vi "Bead Tracking Overlay matches.vi"(7 "Search Rectangle":T4, 8 "error in (no error)":errorcluster, 9 "Bead Tracking Mode":T1, 10 "Matches":T2, 11 "Image":T3) -> (0 "error out":errorcluster, 3 "Image out":T3)   [LabVIEW 2011]
doc: "This VI adds overlays to an image, to show the bead tracking results graphically."
uses:
  <vilib>/vision/Image Controls.llb/IMAQ Image.ctl
  Bead Tracking Matches.ctl
  Bead Tracking Mode.ctl
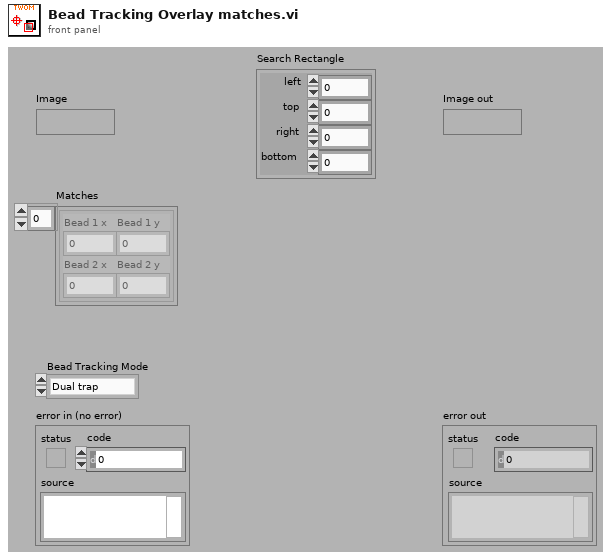
[diagram p1: front panel]
types:
  T1 = typedef "Bead Tracking Mode.ctl" = enum16{"Dual trap", "Q-trap =", "Q-trap ||", "Q-trap X", "Q-trap +", "Dual trap oO", "Single trap", "None"}
  T2 = typedef "Bead Tracking Matches.ctl" = cluster{"Bead 1 x":dbl, "Bead 1 y":dbl, "Bead 2 x":dbl, "Bead 2 y":dbl}[]
  T3 = typedef "IMAQ Image.ctl" = refnum<image>
  T4 = cluster{"left":i16, "top":i16, "right":i16, "bottom":i16}
  T5 = cluster{"Bead 1 x":dbl, "Bead 1 y":dbl, "Bead 2 x":dbl, "Bead 2 y":dbl}
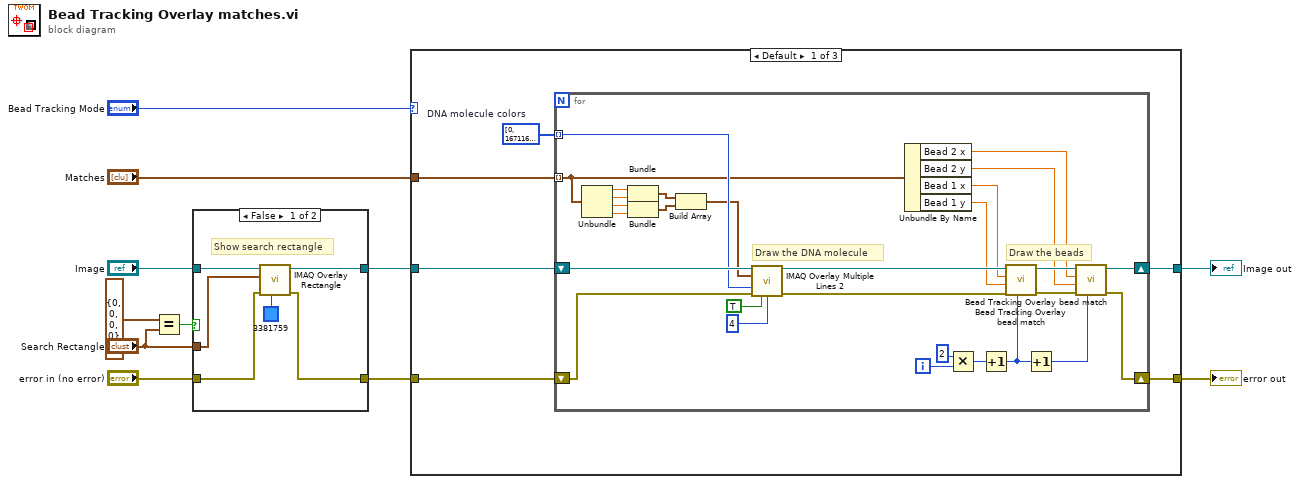
[diagram p0: block diagram]
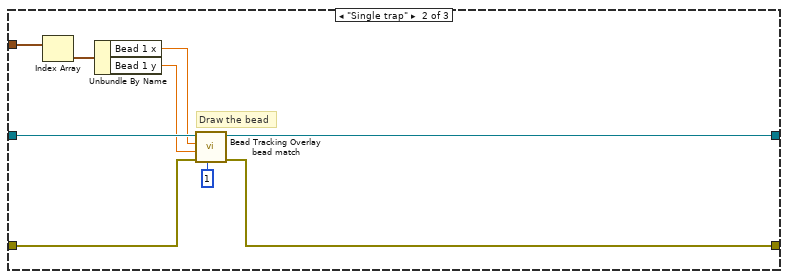
[diagram p2: hidden frame]
diagram:
  n1 = Equal?(x=T4 {"left"=0, "top"=0, "right"=0, "bottom"=0}, y="Search Rectangle") -> (x = y?=w11:bool)
  n2 = case shown="False" w11 {
    tunnel: "Image" -> [w17 w19]
    tunnel: [w16 w19] -> w6
    tunnel: "Search Rectangle" -> [w15 _]
    tunnel: "error in (no error)" -> [w14 w18]
    tunnel: [w12 w18] -> w4
    frame False {
      # "Show search rectangle"
      n3 = call "IMAQ Overlay Rectangle"("Color"=u32 3381759, "error in (no error)"=w14, "Rectangle"=w15, "Image"=w17) -> ("error out"=w12:errorcluster, "Image Out"=w16:T3)  [unwired: 6 in]
    }
    frame True {
      # "We're searching in the whole image, so nothing to show."
    }
  }
  n4 = case shown="Default" "Bead Tracking Mode" {
    tunnel: w6 -> [w25 w62 w64]
    tunnel: [w24 w60 w64] -> w5
    tunnel: w4 -> [w23 w61 w63]
    tunnel: [w22 w57 w63] -> w3
    tunnel: "Matches" -> [w21 w56 _]
    frame Default {
      w20 = u32[] [0, 16711680]  # DNA molecule colors
      n5 = for {
        shift-right: [w27] -> w24
        shift-left: w25 -> [w53]
        shift-right: [w26] -> w22
        shift-left: w23 -> [w28]
        tunnel: w21 -> [w44] mode=indexing
        tunnel: w20 -> [w50] mode=indexing
        i -> [w31]
        # "Draw the beads"
        # "Draw the DNA molecule"
        n6 = Unbundle(w44) -> ("Bead 1 x"=w43:dbl, "Bead 1 y"=w42:dbl, "Bead 2 x"=w41:dbl, "Bead 2 y"=w40:dbl)
        n7 = Bundle("Bead 1 x"=w43, "Bead 1 y"=w42) -> (w39:cluster{"Bead 1 x":dbl, "Bead 1 y":dbl})  [unwired: 1 in]
        n8 = Bundle("Bead 2 x"=w41, "Bead 2 y"=w40) -> (w38:cluster{"Bead 2 x":dbl, "Bead 2 y":dbl})  [unwired: 1 in]
        n9 = Build Array(w39, w38) -> (w37:cluster{"Bead 2 x":dbl, "Bead 2 y":dbl}[])
        n10 = call "IMAQ Overlay Multiple Lines 2"("Image"=w53, "Line End Points"=w37, "Color"=w50, "error in (no error)"=w28, "Maintain Width?"=TRUE, "Width"=u32 4) -> ("Image Out"=w51:T3, "error out"=w29:errorcluster)  [unwired: 8 in]
        n11 = Unbundle By Name(w44) -> ("Bead 2 x"=w46:dbl, "Bead 2 y"=w45:dbl, "Bead 1 x"=w48:dbl, "Bead 1 y"=w49:dbl)
        n12 = Multiply(x=2, y=w31) -> (x*y=w34:i32)
        n13 = Increment(x=w34) -> (x+1=w30:i32)
        n14 = call "Bead Tracking Overlay bead match.vi"("Bead number"=w30, "error in (no error)"=w29, "Y"=w49, "X"=w48, "Image"=w51) -> ("error out"=w47:errorcluster, "Image out"=w52:T3)  [unwired: 5 in]
        n15 = Increment(x=w30) -> (x+1=w32:i32)
        n16 = call "Bead Tracking Overlay bead match.vi"("Bead number"=w32, "error in (no error)"=w47, "Y"=w45, "X"=w46, "Image"=w52) -> ("error out"=w26:errorcluster, "Image out"=w27:T3)  [unwired: 5 in]
      }
    }
    frame "Single trap" {
      # "Draw the bead"
      n17 = Index Array(array=w56) -> (element=w55:T5)  [unwired: 1 in]
      n18 = Unbundle By Name(w55) -> ("Bead 1 x"=w58:dbl, "Bead 1 y"=w59:dbl)
      n19 = call "Bead Tracking Overlay bead match.vi"("Bead number"=1, "error in (no error)"=w61, "Y"=w59, "X"=w58, "Image"=w62) -> ("error out"=w57:errorcluster, "Image out"=w60:T3)  [unwired: 5 in]
    }
    frame "None" {
    }
  }
  "error out" <- w3
  "Image out" <- w5
